vi "SiCenterFinderMercedes.vi"(0 "Operation":enum16{"Manual", "Automatic"}(ring)=enum."Automatic", 1 "Zone":enum16{"ZoneA", "ZoneB", "ZoneC", "ZoneD"}(ring), 2 "Autofocus":T1={"Enable"=TRUE, "InitialStepSize"=0.05, "Tolerance"=0.02, "Abort"=FALSE} {"Tolerance" format="%#_13g"}, 5 "Component":enum16{"Si", "SiOnBP"}(ring), 7 "VisibilityInCamera":enum16{"JoyStick", "AllVisible"}(ring)=enum."AllVisible", 9 "ModuleName":string="T1", 11 "error in (no error)":errorcluster, 12 "Position":enum16{"1", "2"}(ring), 13 "StopJoyStick":bool, 14 "SaveImagesLog":bool=TRUE) -> (4 "Output XYZU":string, 6 "Image":T3(plugin-control), 8 "Image 2":T3[](array[plugin-control]) caption="AllImages", 15 "error out":errorcluster)   [LabVIEW 2019]
uses:
  <vilib>/userDefined/High Color/IMAQdx.ctl
  <vilib>/Analysis/coordinate.llb/2D Cartesian Coordinate Rotation (Scalar).vi
  <vilib>/Analysis/baseanly.llb/Mean (DBL).vi
  Other Models/2010/Motion/AbortSingle.vi
  include/GlobalVariables.vi
  <vilib>/Analysis/NI_AALPro.lvlib
  <vilib>/Analysis/NI_AALBase.lvlib
panel:
  in  "MatchParameters":T2={"Number of Matches Requested"=1, "Minimum Match Score"=500.0, "Angle Ranges"=[{"Start Angle"=0.0, "End Angle"=0.0}]}
  out "OutputFile":string
  out "spreadsheet string 2":string
  out "spreadsheet string":string
  out "SyringeY":dbl format="%#_7g"
  out "SyringeX":dbl format="%#_7g"
  in  "CamToSyringeYoffset":dbl=126.651
  in  "CamToSyringeXoffset":dbl=167.702
  out "FileUsedForFiducials":string
  out "UsedCoordinates":string
  out "CameraGcode":string
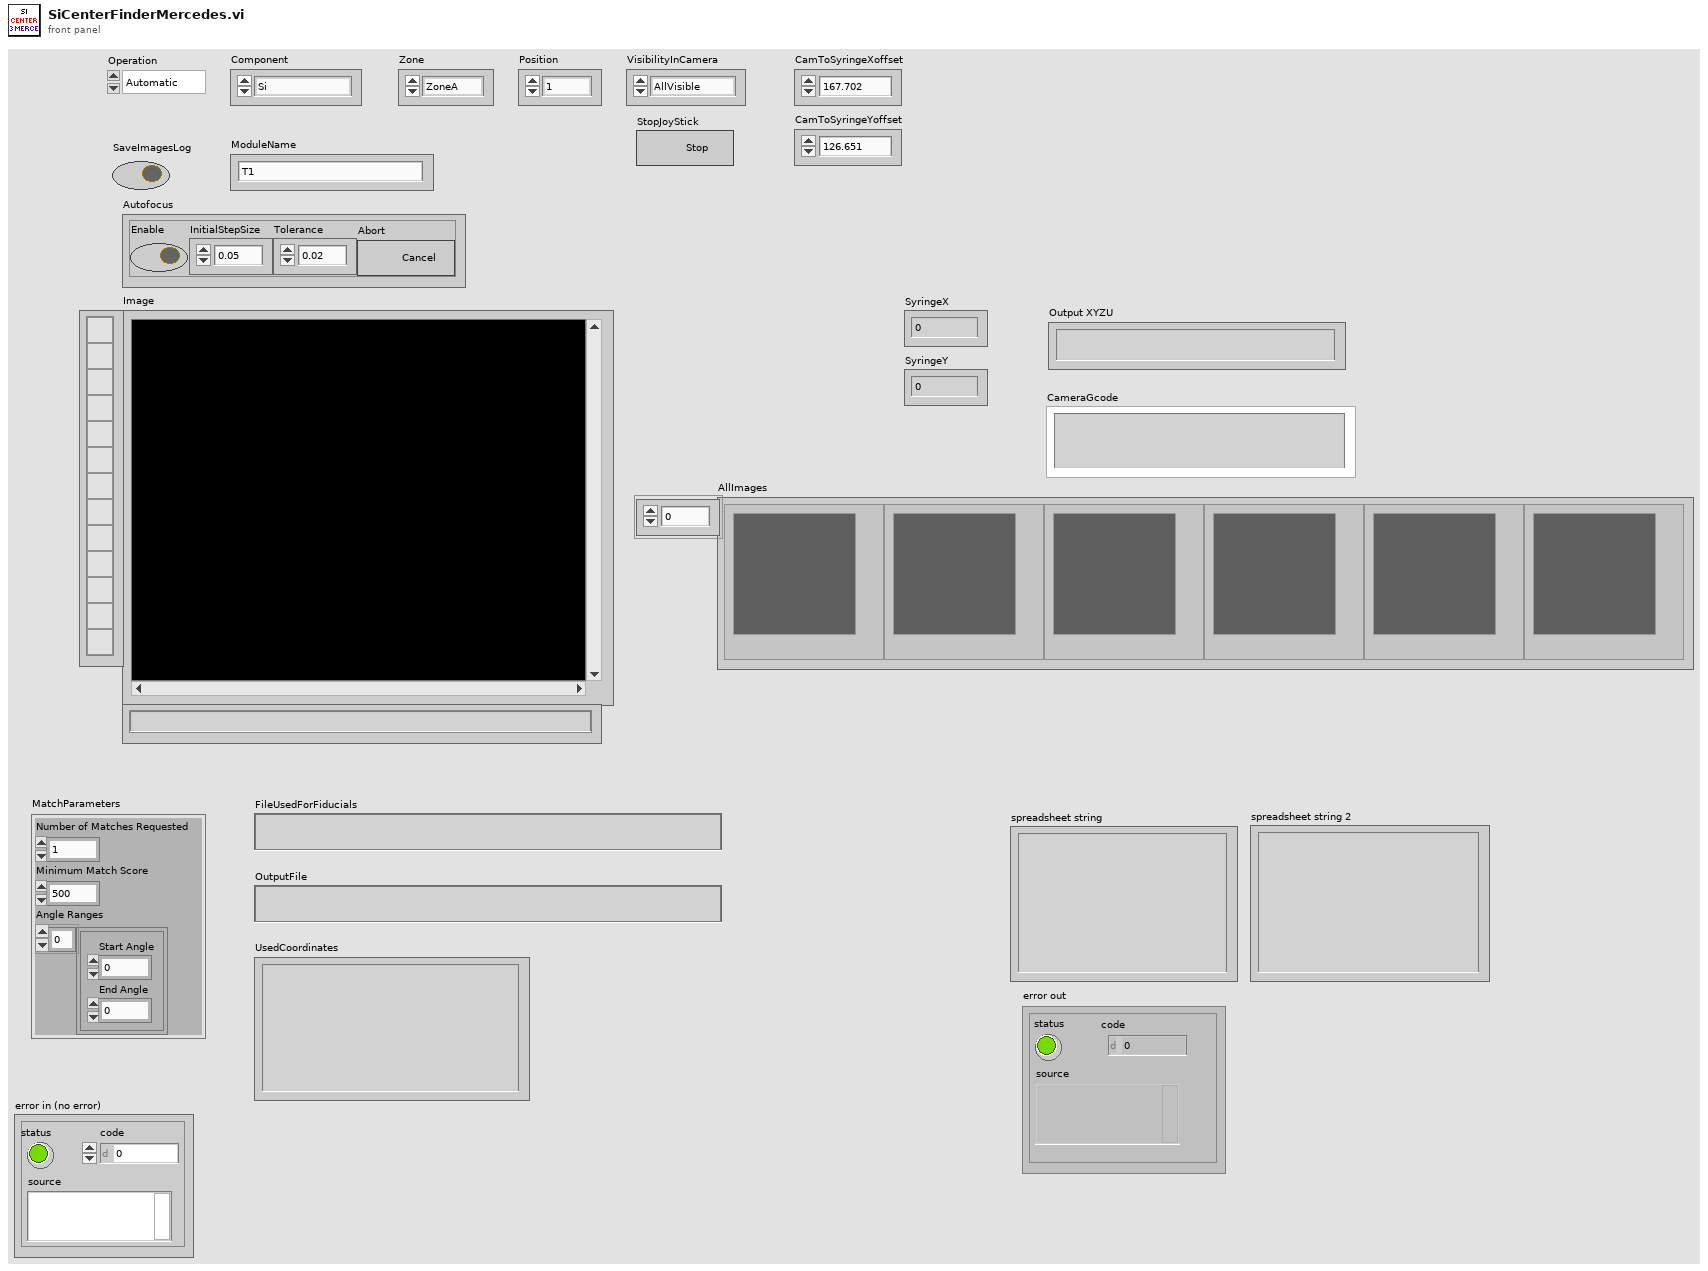
[diagram p1: front panel]
types:
  T1 = cluster{"Enable":bool, "InitialStepSize":dbl, "Tolerance":dbl, "Abort":bool}
  T2 = cluster{"Number of Matches Requested":i32, "Minimum Match Score":sgl, "Angle Ranges":cluster{"Start Angle":sgl, "End Angle":sgl}[]}
  T3 = typedef "IMAQ Image.ctl" = refnum<image>
  T4 = typedef "IMAQdx.ctl" = refnum<k21>
  T5 = typedef "Image Type" = u32
  T6 = typedef "IMAQ Point" = cluster{"X":sgl, "Y":sgl}
  T7 = enum16{"Left Button", "Center Button", "Right Button", "Window Close"}
  T8 = enum16{"open", "replace", "create", "open or create", "replace or create", "replace or create with confirmation"}
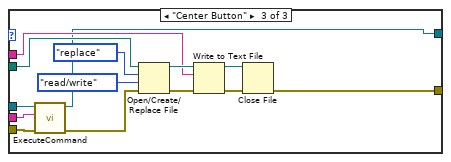
[diagram p4: hidden frame]
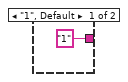
[diagram p5: hidden frame]
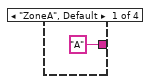
[diagram p6: hidden frame]
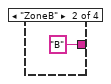
[diagram p7: hidden frame]
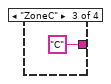
[diagram p8: hidden frame]
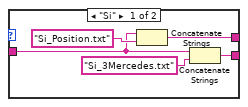
[diagram p9: hidden frame]
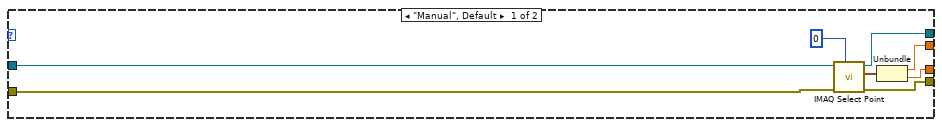
[diagram p10: hidden frame]
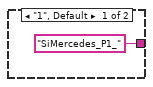
[diagram p11: hidden frame]
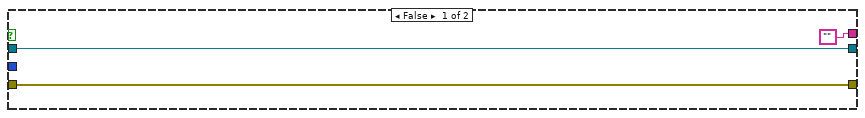
[diagram p12: hidden frame]
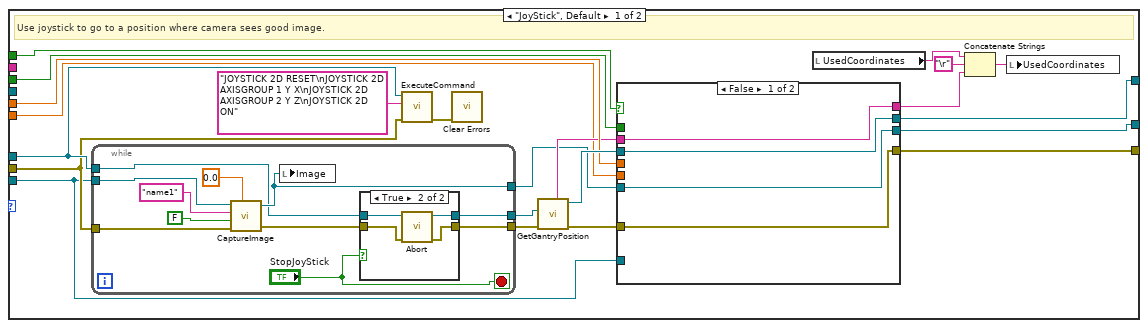
[diagram p13: hidden frame]
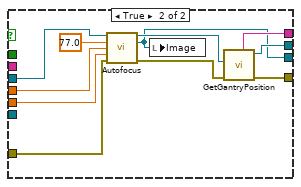
[diagram p14: hidden frame]
diagram:
  w21 = "%f" ("format string")
  w63 = "\t"
  w60 = i16 6 ("width (-)")
  # "Write the XYZU of the baseplate to a text file & move the gantry?"
  # "Prepare to move the gantry to see the center of component in camera."
  # "AllVisble: Assumes that you know the coordinates of all corners (fiducials) well. No need for any adjustments.\nJoyStick: Use joystick at each point to make good image.\nClickMove: Use \"AdjustCamera\" panel and move the gantry stepwise. Click \"Done\" when you're satisfied with the picture."
  n1 = flat-sequence {
    tunnel: [w74] -> w17
    tunnel: w17 -> [w90]
    tunnel: [w89] -> w16
    tunnel: [w88] -> w14
    tunnel: [w87] -> w11
    tunnel: w16 -> [w119]
    tunnel: [w119] -> w15
    tunnel: w14 -> [w118]
    tunnel: [w117] -> w13
    tunnel: [w116] -> w12
    tunnel: w11 -> [w115]
    tunnel: [w115] -> w10
    tunnel: 3 -> [w143]
    tunnel: [w142] -> w23
    tunnel: [w141] -> w22
    tunnel: [w140] -> w69
    tunnel: [w139] -> w3
    tunnel: [w138] -> w41
    tunnel: "VisibilityInCamera" -> [w137]
    tunnel: [w136] -> w26
    tunnel: w15 -> [w135]
    tunnel: w13 -> [w134]
    tunnel: w12 -> [w133]
    tunnel: w10 -> [w132]
    tunnel: [w132] -> w9
    tunnel: [w131] -> w8
    frame #0 {
      n2 = case shown="\"ZoneD\"" "Zone" {
        tunnel: ["A" "B" "C" "D"] -> w78
        frame "ZoneA", Default {
        }
        frame "ZoneB" {
        }
        frame "ZoneC" {
        }
        frame "ZoneD" {
        }
      }
      n3 = case shown="\"2\"" "Position" {
        tunnel: ["1" "2"] -> w79
        frame "1", Default {
        }
        frame "2" {
        }
      }
      n4 = Concatenate Strings(w78, w79, "_" ("string")) -> (w74:string)
      "UsedCoordinates" <- ""
    }
    frame #1 {
      n5 = Concatenate Strings("C:\\Users\\TTUHEP\\Documents\\LabVIEW\\GantryPrograms\\", "Configs\\" ("string"), w90) -> (w97:string)
      n6 = case shown="\"SiOnBP\"" "Component" {
        tunnel: w97 -> [w106 w111]
        tunnel: [w108 w113] -> w100
        tunnel: [w105 w110] -> w87
        frame "Si" {
          n7 = Concatenate Strings(w106, "Si_Position.txt") -> (w105:string)
          n8 = Concatenate Strings(w106, "Si_3Mercedes.txt") -> (w108:string)
        }
        frame "SiOnBP" {
          n9 = Concatenate Strings(w111, "BP_Position.txt") -> (w110:string)
          n10 = Concatenate Strings(w111, "SiOnBP_3Mercedes.txt") -> (w113:string)
        }
      }
      "FileUsedForFiducials" <- w100
      "OutputFile" <- w87
      n11 = String To Path(string=w100) -> (path=w98:path)
      n12 = Concatenate Strings("This file does not exist:" ("ErrorMessage"), w100) -> (w101:string)
      n13 = call <vilib>:"Check if File or Folder Exists.vi"("error in (no error)"="error in (no error)", "path"=w98) -> ("error out"=w99:errorcluster, "file or folder exists?"=w102:bool, "dup path"=w89:path)  [unwired: 7 in]
      n14 = Not(x=w102) -> (.not. x?=w103:bool)
      n15 = call "AddError.vi"("NoErrorMessage"="InFile OK", "ErrorMessage"=w101, "error in"=w99, "code"=-995, "Error?"=w103) -> ("Error out"=w88:errorcluster)  [unwired: 6 in]
    }
    frame #2 {
      # "Set the size of the window while selecting the point."
      n16 = call "IMAQ WindSize"("Scrollbars? (N)"=TRUE, "Width & Height"=cluster{"Width":i32, "Height":i32} {"Width"=1333, "Height"=1000}, "Window Number"=0) -> ()  [unwired: 3 in, 3 out]
      n17 = call "Connect.vi"("error in (no error)"=w118) -> ("error out"=w121:errorcluster, "controller"=w122:refnum<k24>)  [unwired: 9 in]
      n18 = call "ExecuteCommand.vi"("error in (no error)"=w121, "Command Code"="G90\nG1 Z0 F100", "controller in"=w122) -> ("error out"=w117:errorcluster, "controller out"=w116:refnum<k24>)  [unwired: 6 in, 1 out]
    }
    frame #3 {
      n19 = local read "Autofocus"() -> (w130:T1)
      n20 = Unbundle By Name(w130) -> ("Enable"=w129:bool, "Abort"=w128:bool, "InitialStepSize"=w126:dbl, "Tolerance"=w127:dbl)
      n21 = for {
        N: w143 -> [_]
        tunnel: w134 -> [w178]
        tunnel: w133 -> [w202]
        tunnel: w135 -> [w179]
        tunnel: [w176] -> w142 mode=indexing
        tunnel: [w175] -> w141 mode=indexing
        tunnel: [w174] -> w140 mode=indexing
        tunnel: [w160] -> w139 mode=indexing
        tunnel: [w171] -> w138
        tunnel: w137 -> [w170]
        tunnel: w128 -> [w168]
        tunnel: w129 -> [w167]
        tunnel: w126 -> [w166]
        tunnel: [w162] -> w136
        tunnel: [w157] -> w131 mode=indexing
        tunnel: w127 -> [w145]
        i -> [w146]
        w147 = T5 6 items=["Grayscale (U8)", "Grayscale (I16)", "Grayscale (SGL)", "Complex (CSG)", "RGB (U32)", "HSL (U32)", "RGB (U64)", "Grayscale (U16)"] ("Image Type")
        w159 = "name1" ("ImageName")
        w198 = T4 "cam1" ("Camera")
        # "Array of XY cluser"
        # "Z array"
        # "Y array"
        # "X array"
        # "Read text file line by line. Each line contains X,Y,Z coordinates for the gantry."
        n22 = call "GetArrayFmTxtFile.vi"("error in"=w178, "LineNo."=w146, "TextFile"=w179) -> ("error out"=w177:errorcluster, "Array"=w209:dbl[])
        n23 = Index Array(array=w209, index=0) -> (element=w204:dbl)
        n24 = Index Array(array=w209, index=1) -> (element=w203:dbl)
        n25 = Index Array(array=w209, index=2) -> (element=w205:dbl)
        n26 = call "Move.vi"("X"=w204, "Absolute"=TRUE, "Y"=w203, "Z"=w205, "SpeedXY (mm/s)"=100.0, "SpeedZ (mm/s)"=100.0, "Move Z first"=FALSE) -> ("Position Gcode"=w201:string)  [unwired: 8 in]
        n27 = call "ExecuteCommand.vi"("error in (no error)"=w177, "Command Code"=w201, "controller in"=w202) -> ("error out"=w200:errorcluster, "controller out"=w197:refnum<k24>)  [unwired: 6 in, 1 out]
        n28 = call "CaptureImage.vi"("Camera"=w198, "Rotate (degrees)"=sgl 0.0, "ImageName"=w159, "Draw50MicroCircleAtCenter"=FALSE, "error in (no error)"=w200) -> ("Image"=w169:T3, "error out"=w196:errorcluster)  [unwired: 2 in]
        n29 = local write "Image"(w169) -> ()
        n30 = case shown="\"AllVisible\"" w170 {
          tunnel: w198 -> [w280 w332]
          tunnel: w197 -> [w296 w346]
          tunnel: w196 -> [w294 w347]
          tunnel: [w276 w334] -> w164
          tunnel: [w283 w340] -> w184
          tunnel: [w284 w338] -> w183
          tunnel: w169 -> [_ w333]
          tunnel: w168 -> [w287 w344]
          tunnel: w167 -> [w282 w345]
          tunnel: w166 -> [w281 w343]
          tunnel: w159 -> [_ w331]
          tunnel: w145 -> [w278 w330]
          frame "JoyStick", Default {
            # "Use joystick to go to a position where camera sees good image."
            n31 = while {
              tunnel: w280 -> [w322]
              tunnel: [w319] -> w277
              tunnel: w296 -> [w318]
              tunnel: [w315] -> w292
              tunnel: [w314] -> w293
              tunnel: w294 -> [w313]
              stop <- "StopJoyStick" stop-if-true
              n32 = call "CaptureImage.vi"("Camera"=w322, "Rotate (degrees)"=sgl 0.0, "ImageName"="name1", "Draw50MicroCircleAtCenter"=FALSE, "error in (no error)"=w313) -> ("Image"=w319:T3, "error out"=w316:errorcluster)  [unwired: 2 in]
              n33 = local write "Image"(w319) -> ()
              n34 = case shown="True" "StopJoyStick" {
                tunnel: w318 -> [w325 w329]
                tunnel: w316 -> [w324 w328]
                tunnel: [w324 w327] -> w315
                tunnel: [w325 w326] -> w314
                frame False {
                }
                frame True {
                  n35 = call-poly "Abort.vi"("error in (no error)"=w328, "controller in"=w329) -> ("error out"=w327:errorcluster, "controller out"=w326:refnum<k24>)  [unwired: 8 in]
                }
              }
            }
            n36 = call "ExecuteCommand.vi"("error in (no error)"=w294, "Command Code"="JOYSTICK 2D RESET\nJOYSTICK 2D AXISGROUP 1 Y X\nJOYSTICK 2D AXISGROUP 2 Y Z\nJOYSTICK 2D ON", "controller in"=w296) -> ("error out"=w295:errorcluster)  [unwired: 6 in, 2 out]
            n37 = call <vilib>:"Clear Errors.vi"("error in (no error)"=w295) -> ()  [unwired: 5 in, 2 out]
            n38 = call "GetGantryPosition.vi"("error in (no error)"=w292, "Controller In"=w293) -> ("error out"=w288:errorcluster, "controller out"=w286:refnum<k24>, "Position_XYZ"=w279:string)  [unwired: 3 in, 4 out]
            n39 = case shown="False" w282 {
              tunnel: w288 -> [w301 w312]
              tunnel: w287 -> [_ _]
              tunnel: w286 -> [w299 w306]
              tunnel: [w300 w310] -> w285
              tunnel: [w301 w309] -> w284
              tunnel: [w299 w308] -> w283
              tunnel: w279 -> [w300 _]
              tunnel: w281 -> [_ w304]
              tunnel: w280 -> [_ _]
              tunnel: w278 -> [_ w303]
              tunnel: w277 -> [w298 _]
              tunnel: [w298 w302] -> w276
              frame False {
              }
              frame True {
                n40 = call "Autofocus.vi"("controller in"=w306, "SafeMaxZ"=77.0, "InitialStepSize"=w304, "Tolerance"=w303, "error in (no error)"=w312) -> ("controller out"=w311:refnum<k24>, "Image"=w302:T3, "error out"=w307:errorcluster)  [unwired: 6 in, 2 out]
                n41 = local write "Image"(w302) -> ()
                n42 = call "GetGantryPosition.vi"("error in (no error)"=w307, "Controller In"=w311) -> ("error out"=w309:errorcluster, "controller out"=w308:refnum<k24>, "Position_XYZ"=w310:string)  [unwired: 3 in, 4 out]
              }
            }
            n43 = local read "UsedCoordinates"() -> (w290:string)
            n44 = Concatenate Strings(w290, "\r", w285) -> (w291:string)
            n45 = local write "UsedCoordinates"(w291) -> ()
          }
          frame "AllVisible" {
            # "No need to move gantry to take a good pic."
            n46 = case shown="True" w345 {
              tunnel: w344 -> [_ _]
              tunnel: [w350 w352] -> w339
              tunnel: [w349 w358] -> w341
              tunnel: w347 -> [w350 w355]
              tunnel: w346 -> [w349 w357]
              tunnel: w343 -> [_ w354]
              tunnel: [w348 w351] -> w334
              tunnel: w333 -> [w348 _]
              tunnel: w332 -> [_ _]
              tunnel: w331 -> [_ _]
              tunnel: w330 -> [_ w353]
              frame False {
              }
              frame True {
                n47 = call "Autofocus.vi"("controller in"=w357, "SafeMaxZ"=77.0, "InitialStepSize"=w354, "Tolerance"=w353, "error in (no error)"=w355) -> ("controller out"=w358:refnum<k24>, "Image"=w351:T3, "error out"=w352:errorcluster)  [unwired: 6 in, 2 out]
                n48 = local write "Image"(w351) -> ()
              }
            }
            n49 = local read "UsedCoordinates"() -> (w336:string)
            n50 = call "GetGantryPosition.vi"("error in (no error)"=w339, "Controller In"=w341) -> ("error out"=w338:errorcluster, "controller out"=w340:refnum<k24>, "Position_XYZ"=w337:string)  [unwired: 3 in, 4 out]
            n51 = Concatenate Strings(w336, "\r", w337) -> (w335:string)
            n52 = local write "UsedCoordinates"(w335) -> ()
          }
        }
        n53 = case shown="\"Automatic\"" "Operation" {
          tunnel: [w218 w244] -> w192
          tunnel: [w217 w243] -> w191
          tunnel: [w216 w242] -> w190
          tunnel: w183 -> [w215 w239]
          tunnel: w164 -> [w214 w246]
          tunnel: [w213 w226] -> w156
          tunnel: w146 -> [_ w224]
          frame "Manual", Default {
            n54 = call "IMAQ Select Point"("Window Number (0...15)"=0, "error in (no error)"=w215, "Image In"=w214) -> ("error out"=w216:errorcluster, "Point"=w219:T6, "Image Out (duplicate)"=w213:T3)  [unwired: 5 in, 1 out]
            n55 = Unbundle(w219) -> ("X"=w218:sgl, "Y"=w217:sgl)
          }
          frame "Automatic" {
            w237 = ""
            n56 = local read "Position"() -> (w240:enum16{"1", "2"})
            n57 = case shown="\"2\"" w240 {
              tunnel: ["SiMercedes_P1_" "SiMercedes_P2_"] -> w222
              frame "1", Default {
              }
              frame "2" {
              }
            }
            n58 = Number To Decimal String(number=w224) -> (decimal integer string=w223:string)  [unwired: 1 in]
            n59 = Concatenate Strings("Could not parse/find this template file for pattern recognition:" ("ErrorMessage"), w222) -> (w232:string)
            n60 = Concatenate Strings(w222, w223) -> (w221:string)
            n61 = call "JSONfileReader.vi"("error in"=w239, "Variant"=w237, "ItemName"=w221, "FileIn"=path "C:/Users/TTUHEP/Documents/LabVIEW/GantryPrograms/Configs/PatternRecognTemplateMaps.json" ("PatterRecognTemplateMap")) -> ("error out"=w229:errorcluster, "Data"=w238:variant, "Found"=w235:bool)
            n62 = Not(x=w235) -> (.not. x?=w234:bool)
            n63 = Variant To Data(error in=w229, type=w237, Variant=w238) -> (data=w236:string, error out=w228:errorcluster)
            n64 = call "AddError.vi"("NoErrorMessage"="Template file name found from json.", "ErrorMessage"=w232, "error in"=w228, "code"=-902, "Error?"=w234) -> ("Error out"=w227:errorcluster)  [unwired: 6 in]
            n65 = call "PatternRecognition.vi"("error in (no error)"=w227, "MatchParameters"="MatchParameters", "ImageIn"=w246, "TemplateFileName"=w236) -> ("error out"=w242:errorcluster, "Position"=w245:cluster{"x":sgl, "y":sgl}, "ImageFoundPattern"=w226:T3)  [unwired: 2 in, 2 out]
            n66 = Unbundle(w245) -> ("x"=w244:sgl, "y"=w243:sgl)
          }
        }
        n67 = Number To Decimal String(number=w146) -> (decimal integer string=w155:string)  [unwired: 1 in]
        n68 = Concatenate Strings("imgTemp" ("string"), w155) -> (w152:string)
        n69 = call "GetPixelToGantryRelPosition.vi"("error in (no error)"=w190, "PixelY"=w191, "PixelX"=w192) -> ("error out"=w150:errorcluster, "YmmRelGH"=w188:dbl, "XmmRelGH"=w189:dbl)
        n70 = call "IMAQ Create"("Image Name"=w152, "Image Type"=w147, "error in (no error)"=w150) -> ("New Image"=w151:T3, "error out"=w149:errorcluster)  [unwired: 2 in]
        n71 = call "IMAQ Copy"("error in (no error)"=w149, "Image Dst"=w151, "Image Src"=w156) -> ("error out"=w148:errorcluster, "Image Dst Out"=w153:T3)  [unwired: 3 in]
        n72 = Build Array(w153) -> (w157:T3[])
        n73 = flat-sequence {
          tunnel: w148 -> [w267]
          tunnel: [w267] -> w194
          tunnel: w184 -> [w266]
          tunnel: [w266] -> w193
          tunnel: [w275] -> w161
          tunnel: [w274] -> w187
          tunnel: [w273] -> w186
          tunnel: [w272] -> w171
          tunnel: [w271] -> w185
          tunnel: w194 -> [w270]
          tunnel: w193 -> [w269]
          frame #0 {
            n74 = Wait (ms)(milliseconds to wait=u32 1000) -> ()  [unwired: 1 out]
          }
          frame #1 {
            n75 = call "GetGantryPosition.vi"("error in (no error)"=w270, "Controller In"=w269) -> ("error out"=w275:errorcluster, "Position Y"=w274:dbl, "Position X"=w273:dbl, "controller out"=w272:refnum<k24>, "Position Z"=w271:dbl)  [unwired: 3 in, 2 out]
          }
        }
        n76 = Add(x=w189, y=w186) -> (x+y=w182:dbl)
        n77 = Add(x=w188, y=w187) -> (x+y=w181:dbl)
        n78 = case shown="True" "SaveImagesLog" {
          tunnel: w156 -> [w249 w265]
          tunnel: w146 -> [_ w263]
          tunnel: ["" w255] -> w162
          tunnel: w161 -> [w250 w254]
          tunnel: [w250 w253] -> w160
          tunnel: [w249 w252] -> w144
          frame False {
          }
          frame True {
            w257 = "C:\\Users\\TTUHEP\\Documents\\LabVIEW\\GantryPrograms\\LogFiles\\CalibrationData\\"
            n79 = Number To Decimal String(number=w263) -> (decimal integer string=w261:string)  [unwired: 1 in]
            n80 = Concatenate Strings(w257, "ModuleName") -> (w255:string)
            n81 = Concatenate Strings(w257, "ModuleName", "Image" ("string"), w261, ".png" ("string")) -> (w259:string)
            n82 = String To Path(string=w259) -> (path=w258:path)
            n83 = call-poly "IMAQ Write File 2"("error in (no error)"=w254, "Image Quality"=u32 1000, "File Path"=w258, "Image"=w265) -> ("error out"=w253:errorcluster, "Image Out (duplicate)"=w252:T3)  [unwired: 6 in]
          }
        }
        "Image" <- w144
        n84 = call-poly <vilib>:"2D Cartesian Coordinate Rotation.vi"("theta"=0.0, "y"=w181, "x"=w182) -> ("y out"=w172:dbl, "x out"=w173:dbl)  [unwired: 6 in, 1 out]
        n85 = global write "GlobalVariables.vi" "Image"(w144) -> ()
        n86 = Build Array(w172) -> (w175:dbl[])
        n87 = Build Array(w173) -> (w176:dbl[])
        n88 = Build Array(w185) -> (w174:dbl[])
      }
    }
  }
  n89 = Array To Spreadsheet String(array=w22, 3:w21) -> (spreadsheet string=→"spreadsheet string 2":string)  [unwired: 1 in]
  n90 = Array To Spreadsheet String(array=w23, 3:w21) -> (spreadsheet string=→"spreadsheet string":string)  [unwired: 1 in]
  n91 = String To Path(string=w9) -> (path=w18:path)
  n92 = Index Array(array=w8, index (col)=0 ("disabled index (col)")) -> (element=→"Image 2":T3[])  [unwired: 1 in]
  n93 = Index Array "Z"(array=w69, index (col)=0 ("disabled index (col)")) -> (element=w68:dbl[])  [unwired: 1 in]
  n94 = Index Array "Y"(array=w22, index (col)=0 ("disabled index (col)")) -> (element=w66:dbl[])  [unwired: 1 in]
  n95 = Index Array "X"(array=w23, index (col)=0 ("disabled index (col)")) -> (element=w67:dbl[])  [unwired: 1 in]
  n96 = formula code="float64 m1 = 0.0, x = 0.0, y = 0.0;\nfloat64 orientn = 0.0, angl1 = 0.0;\n\nm1 = (yin[1] - yin[0]) / (xin[1] - xin[0]);\nangl1 = (atan(m1)*180.0/3.14159);\norientn = angl1;\n\nx = xin[2];\ny = yin[2];"("xin"=w67, "yin"=w66) -> ("orientn"=w42:dbl, "x"=w5:dbl, "y"=w4:dbl)
  n97 = call-poly <vilib>:"Mean.vi"("X"=w68) -> ("mean"=w43:dbl)  [unwired: 1 out]
  n98 = Number To Fractional String(number=w5, precision (6)=w60) -> (F-format string=w65:string)  [unwired: 2 in]
  n99 = Number To Fractional String(number=w4, precision (6)=w60) -> (F-format string=w64:string)  [unwired: 2 in]
  n100 = Number To Fractional String(number=w43, precision (6)=w60) -> (F-format string=w59:string)  [unwired: 2 in]
  n101 = call "CameraXYusingGantryHeadXY.vi"("GantryY"=w4, "GantryX"=w5) -> ("CamY"=w32:dbl, "CamX"=w34:dbl)
  n102 = Number To Fractional String(number=w42, precision (6)=i16 4 ("width (-)")) -> (F-format string=w61:string)  [unwired: 2 in]
  n103 = call "Move.vi"("X"=w34, "Absolute"=TRUE, "Y"=w32, "Z"=w43, "SpeedXY (mm/s)"=100.0, "SpeedZ (mm/s)"=50.0, "Move Z first"=TRUE) -> ("Position Gcode"=w46:string)  [unwired: 8 in]
  "CameraGcode" <- w46
  n104 = Add(x="CamToSyringeYoffset", y=w32) -> (x+y=→"SyringeY":dbl)
  n105 = Concatenate Strings(w65, w63, w64, w63, w59, w63, w61, "\r") -> (w57:string)
  "Output XYZU" <- w57
  n106 = Add(x="CamToSyringeXoffset", y=w34) -> (x+y=→"SyringeX":dbl)
  n107 = Concatenate Strings("Overwrite/Append ", w57, " to file ", w9, " ?" ("string")) -> (w54:string)
  n108 = call <vilib>:"Three Button Dialog.vi"("Right Button Text (\"Cancel\")"="Do nothing" ("Right Button Text (\"Cancel\")"), "Center Button Text (\"No\")"="Overwrite" ("Left Button Text (\"Yes\")"), "Left Button Text (\"Yes\")"="Append" ("Center Button Text (\"No\")"), "message"=w54) -> ("Which Button?"=w53:T7)  [unwired: 7 in]
  n109 = Merge Errors(w3) -> (w2:errorcluster)
  n110 = case shown="\"Left Button\", Default" w53 {
    tunnel: w57 -> [w372 _ w386]
    tunnel: w18 -> [w371 _ w385]
    tunnel: w2 -> [w370 w378 w384]
    tunnel: w46 -> [w369 _ w383]
    tunnel: w41 -> [w368 w377 w382]
    tunnel: [w359 w378 w379] -> w28
    tunnel: [w367 w377 w381] -> w45
    frame "Left Button", Default {
      n111 = call "ExecuteCommand.vi"("error in (no error)"=w370, "Command Code"=w369, "controller in"=w368) -> ("error out"=w360:errorcluster, "controller out"=w367:refnum<k24>)  [unwired: 6 in, 1 out]
      n112 = Open/Create/Replace File(file path (use dialog)=w371, error in=w360, operation (0:open)=T8."open or create", access (0:read/write)=enum16{"read/write", "read-only", "write-only"}."read/write") -> (refnum out=w364:refnum<file>, error out=w362:errorcluster)  [unwired: 2 in, 1 out]
      n113 = Set File Position(offset (in bytes) (0)=i64 0, refnum=w364, from (0:start)=enum16{"start", "end", "current"}."end", error in=w362) -> (refnum out=w363:refnum<file>, error out=w361:errorcluster)
      n114 = Write to Text File(file (use dialog)=w363, text=w372, error in=w361) -> (refnum out=w373:refnum<file>, error out=w374:errorcluster)  [unwired: 1 in, 1 out]
      n115 = Close File(refnum=w373, error in=w374) -> (error out=w359:errorcluster)  [unwired: 1 out]
    }
    frame "Right Button" {
    }
    frame "Center Button" {
      n116 = call "ExecuteCommand.vi"("error in (no error)"=w384, "Command Code"=w383, "controller in"=w382) -> ("error out"=w380:errorcluster, "controller out"=w381:refnum<k24>)  [unwired: 6 in, 1 out]
      n117 = Open/Create/Replace File(file path (use dialog)=w385, error in=w380, operation (0:open)=T8."replace", access (0:read/write)=enum16{"read/write", "read-only", "write-only"}."read/write") -> (refnum out=w392:refnum<file>, error out=w389:errorcluster)  [unwired: 2 in, 1 out]
      n118 = Write to Text File(file (use dialog)=w392, text=w386, error in=w389) -> (refnum out=w387:refnum<file>, error out=w388:errorcluster)  [unwired: 1 in, 1 out]
      n119 = Close File(refnum=w387, error in=w388) -> (error out=w379:errorcluster)  [unwired: 1 out]
    }
  }
  n120 = call "CaptureImage.vi"("Camera"=T4 "cam1", "ImageName"="CurrImage", "Draw50MicroCircleAtCenter"=TRUE, "error in (no error)"=w28) -> ("Image"=w1:T3, "error out"=w27:errorcluster)  [unwired: 3 in]
  n121 = local write "Image"(w1) -> ()
  n122 = global write "GlobalVariables.vi" "Image"(w1) -> ()
  n123 = call "Disconnect.vi"("error in (no error)"=w27, "controller"=w45) -> ("error out"=w24:errorcluster)  [unwired: 9 in]
  n124 = local read "SaveImagesLog"() -> (w29:bool)
  n125 = case shown="True" w29 {
    tunnel: w24 -> [w393 w408]
    tunnel: w26 -> [_ w401]
    tunnel: w1 -> [_ w396]
    tunnel: [w393 w394] -> w25
    frame False {
    }
    frame True {
      n126 = Concatenate Strings(w401, "UsedXYZ.txt") -> (w406:string)
      n127 = local read "UsedCoordinates"() -> (w403:string)
      n128 = Concatenate Strings(w401, "CenterImage.png") -> (w399:string)
      n129 = String To Path(string=w406) -> (path=w405:path)
      n130 = String To Path(string=w399) -> (path=w397:path)
      n131 = Open/Create/Replace File(file path (use dialog)=w405, error in=w408, operation (0:open)=T8."open or create", access (0:read/write)=enum16{"read/write", "read-only", "write-only"}."read/write") -> (refnum out=w404:refnum<file>, error out=w412:errorcluster)  [unwired: 2 in, 1 out]
      n132 = Write to Text File(file (use dialog)=w404, text=w403, error in=w412) -> (refnum out=w402:refnum<file>, error out=w411:errorcluster)  [unwired: 1 in, 1 out]
      n133 = Close File(refnum=w402, error in=w411) -> (error out=w395:errorcluster)  [unwired: 1 out]
      n134 = call-poly "IMAQ Write File 2"("error in (no error)"=w395, "Image Quality"=u32 1000, "File Path"=w397, "Image"=w396) -> ("error out"=w394:errorcluster)  [unwired: 6 in, 1 out]
    }
  }
  "error out" <- w25
